vi "Tektronix.vi"(7 "JPG":refnum<vi>, 10 "queueName":string="PV_script", 11 "Console Reference":refnum<vi>) -> ()   [LabVIEW 2022 SP3]
panel:
  in  "stop":bool
  out "plot":cluster{dbl, dbl, dbl[]}(graph)
  in  "VISA":refnum<visa-resource-name>
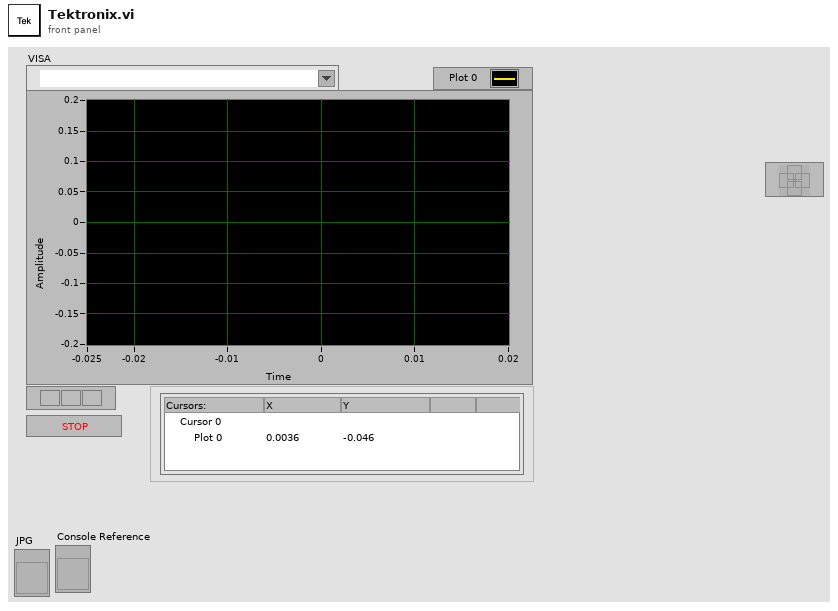
[diagram p1: front panel]
types:
  T1 = enum8{"Enabled", "Disabled", "Disabled and Grayed Out"}
  T2 = cluster{"Xmax":dbl, "Xmin":dbl, "Ymax":dbl, "Ymin":dbl}
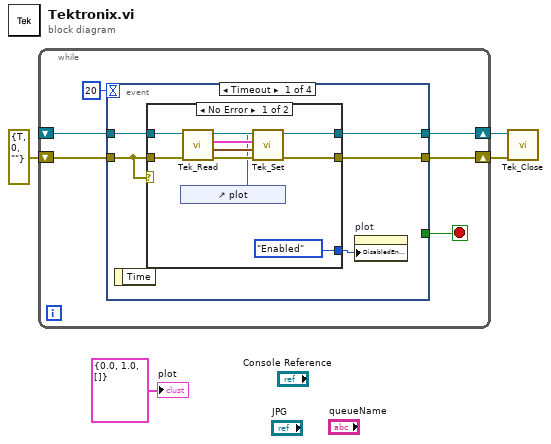
[diagram p0: block diagram]
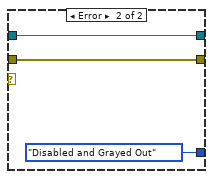
[diagram p2: hidden frame]
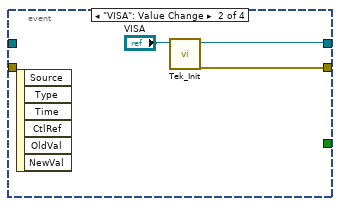
[diagram p3: hidden frame]
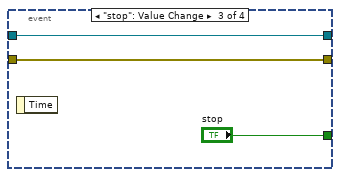
[diagram p4: hidden frame]
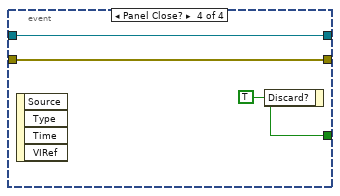
[diagram p5: hidden frame]
diagram:
  n1 = while {
    shift-right: [w10] -> w4
    shift-left: _ -> [w9]
    shift-right: [w7] -> w3
    shift-left: errorcluster {"status"=TRUE, "code"=0, "source"=""} ("error out") -> [w8]
    stop <- w6 stop-if-true
    n2 = event shown="[0] Timeout" {
      selector: _ -> [_ _ _ _]
      dyn-events: _ -> [_ _ _ _]
      timeout: 20 -> [_ _ _ _]
      tunnel: [w15 "VISA" w30 w34] -> w10
      tunnel: w9 -> [w14 _ w30 w34]
      tunnel: w8 -> [w12 _ w29 w33]
      tunnel: [w13 w28 w29 w33] -> w7
      tunnel: [_ _ "stop" w32] -> w6
      event Timeout {
        n3 = event-data() -> ()  [unwired: 1 in, 1 out]
        n4 = case shown="No Error" w12 {
          tunnel: [w23 w26] -> w15
          tunnel: w14 -> [w22 w26]
          tunnel: w12 -> [w21 w25]
          tunnel: [w20 w25] -> w13
          tunnel: [T1."Enabled" ("Disabled") T1."Disabled and Grayed Out" ("Disabled")] -> w11
          frame No Error {
            n5 = control-ref of="plot"() -> (w16:refnum<vi>)
            n6 = call "Tek_Read.vi"("error in (no error)"=w21, "VISA Refnum in"=w22) -> ("error out"=w20:errorcluster, "range"=w17:T2, "Scope"=w18:cluster{dbl, dbl, dbl[]}, "VISA Refnum out"=w23:refnum<visa-resource-name>)  [unwired: 6 in]
            n7 = call "Tek_Set.vi"("error in (no error)"=w20, "range"=w17, "Scope"=w18, "plot"=w16) -> ()  [unwired: 8 in]
          }
          frame Error {
          }
        }
        n8 = property on="plot" class="WFGraph (strict)"("DisabledEnum"=w11) -> ()  [unwired: 2 in, 2 out]
      }
      event "VISA": Value Change {
        n9 = event-data() -> ()  [unwired: 1 in, 6 out]
        n10 = call "Tek_Init.vi"("VISA"="VISA") -> ("error out"=w28:errorcluster)  [unwired: 9 in, 1 out]
      }
      event "stop": Value Change {
        n11 = event-data() -> ()  [unwired: 1 in, 1 out]
      }
      event Panel Close? {
        w32 = TRUE ("Discard?")
        n12 = event-data() -> ()  [unwired: 1 in, 4 out]
        n13 = event-data("Discard?"=w32) -> ()  [unwired: 1 in, 1 out]
      }
    }
  }
  n14 = call "Tek_Close.vi"("error in (no error)"=w3, "VISA Refnum in"=w4) -> ()  [unwired: 10 in]
  "plot" <- cluster{dbl, dbl, dbl[]} {0.0, 1.0, []} ("plot")
